vi "Get Conversion Buffers.vi"(8 "error in (no error)":errorcluster, 10 "inline?":bool, 11 "Transfer in":refnum<class "Transfer.lvclass">) -> (0 "error out":errorcluster, 1 "converted Buffer":refnum<class "Buffer.lvclass">, 2 "unconverted Buffer":refnum<class "Buffer.lvclass">, 3 "Transfer out":refnum<class "Transfer.lvclass">)   [LabVIEW 2017, in "DSF Core.lvlib" / "Transfer.lvclass"]
uses:
  Transfer.lvclass
  Buffer/Buffer.lvclass
  Transfer.lvclass/Transfer.ctl
  Buffer/Buffers.lvclass
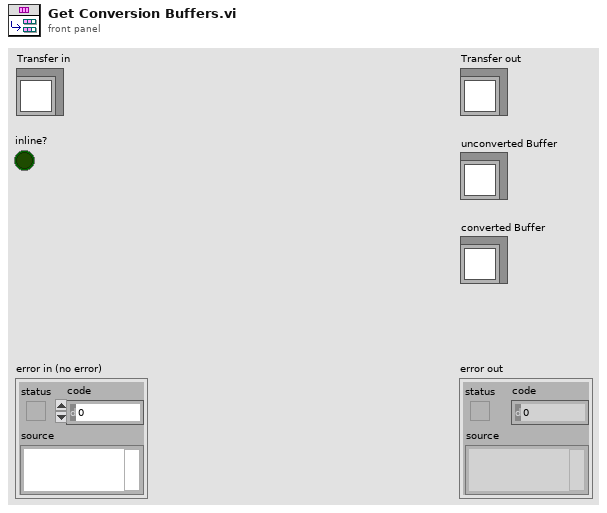
[diagram p1: front panel]
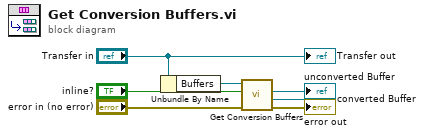
[diagram p0: block diagram]
diagram:
  n1 = Unbundle By Name("Transfer in") -> ("Buffers"=w6:refnum<class "Buffers.lvclass">)
  n2 = call "Get Conversion Buffers.vi"("error in (no error)"="error in (no error)", "inline?"="inline?", "Buffers in"=w6) -> ("error out"=→"error out":errorcluster, "converted Buffer"=→"converted Buffer":refnum<class "Buffer.lvclass">, "unconverted Buffer"=→"unconverted Buffer":refnum<class "Buffer.lvclass">)  [unwired: 5 in, 1 out]
  "Transfer out" <- "Transfer in"
